vi "StationMeteo.vi"() -> ()   [LabVIEW 2018]
uses:
  <vilib>/Instr/_visa.llb/VISA Configure Serial Port (Instr).vi
panel:
  out "Nombre mesures":dbl
  out "Moyenne 3":dbl
  out "Maximum 3":dbl
  out "Minimum 3":dbl
  out "Moyenne 2":dbl
  out "Maximum 2":dbl
  out "Minimum 2":dbl
  out "Moyenne":dbl
  out "Maximum":dbl
  out "Minimum":dbl
  in  "Nom du fichier":string
  in  "Seléctionner un répertoire":bool
  out "Répertoire":path
  in  "Export valeurs":bool
  out "?":bool
  out "CSV string":string
  in  "En marche":bool
  out "Waveform Graph":dbl[](graph)
  out "boucle":dbl[](array[numeric])
  out "temperature test":dbl[](array[numeric])
  out "XY Graph":T1(graph)
  out "Humidité":dbl(graph)
  out "Pression":dbl(graph)
  out "Température":dbl(graph)
  out "Humidité temps réel":dbl
  out "Pression temps réel":dbl
  out "Température temps réel":dbl
  out "Chaîne":string
  in  "stop":bool
  in  "Nom de ressource VISA":refnum<visa-resource-name>
  # "1. Brancher la carte Arduino sur un port USB\n2. Choisir le port COM de la carte dans la liste déroulante \"Nom de ressource VISA\"\n3. Lancer le programme"
  # "Contrôles de la station météo"
  # "Valeurs particulières"
  # "Valeurs particulières"
  # "Sauvegardes des mesures en CSV"
  # "Valeurs particulières"
  # ".csv"
  # "Fichier global"
  # "Fichier séparé"
  # "Fichier séparé rajoute un -numéro à la fin \nnom de fichier. Ex: releve-5.csv\nFichier global rajoute un -global à la fin \ndu nom de fichier. Ex: releve-global.csv"
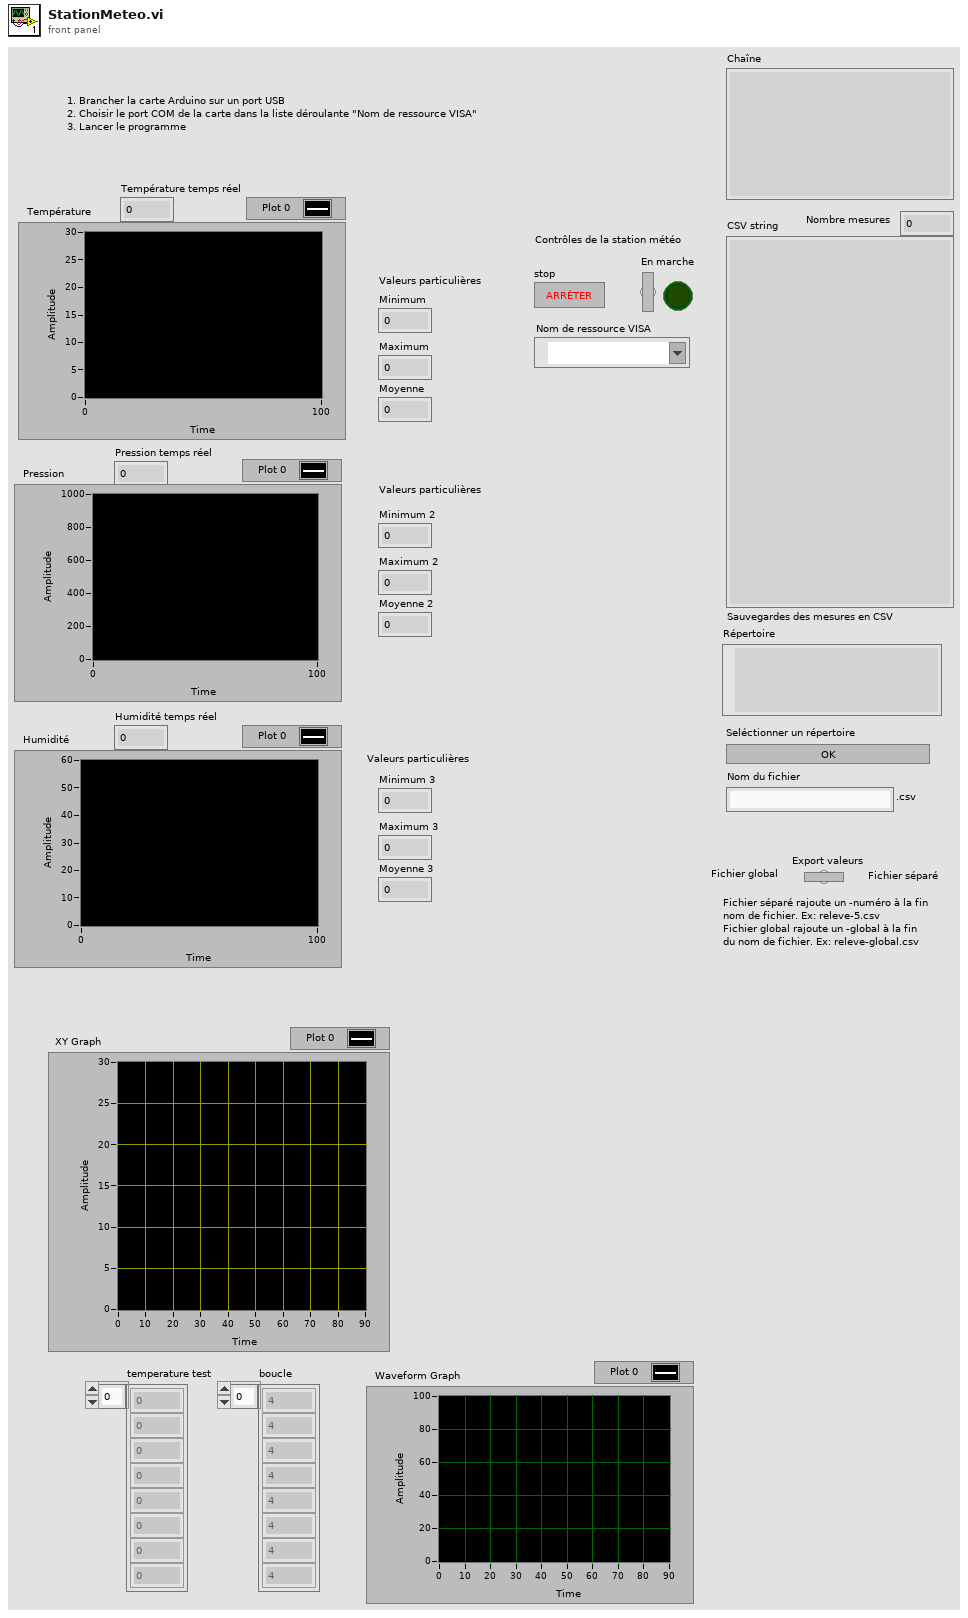
[diagram p1: front panel]
types:
  T1 = cluster{"temperature test":dbl[], "boucle":dbl[]}
  T2 = cluster{"boucle":dbl[], "temperature test":dbl[]}
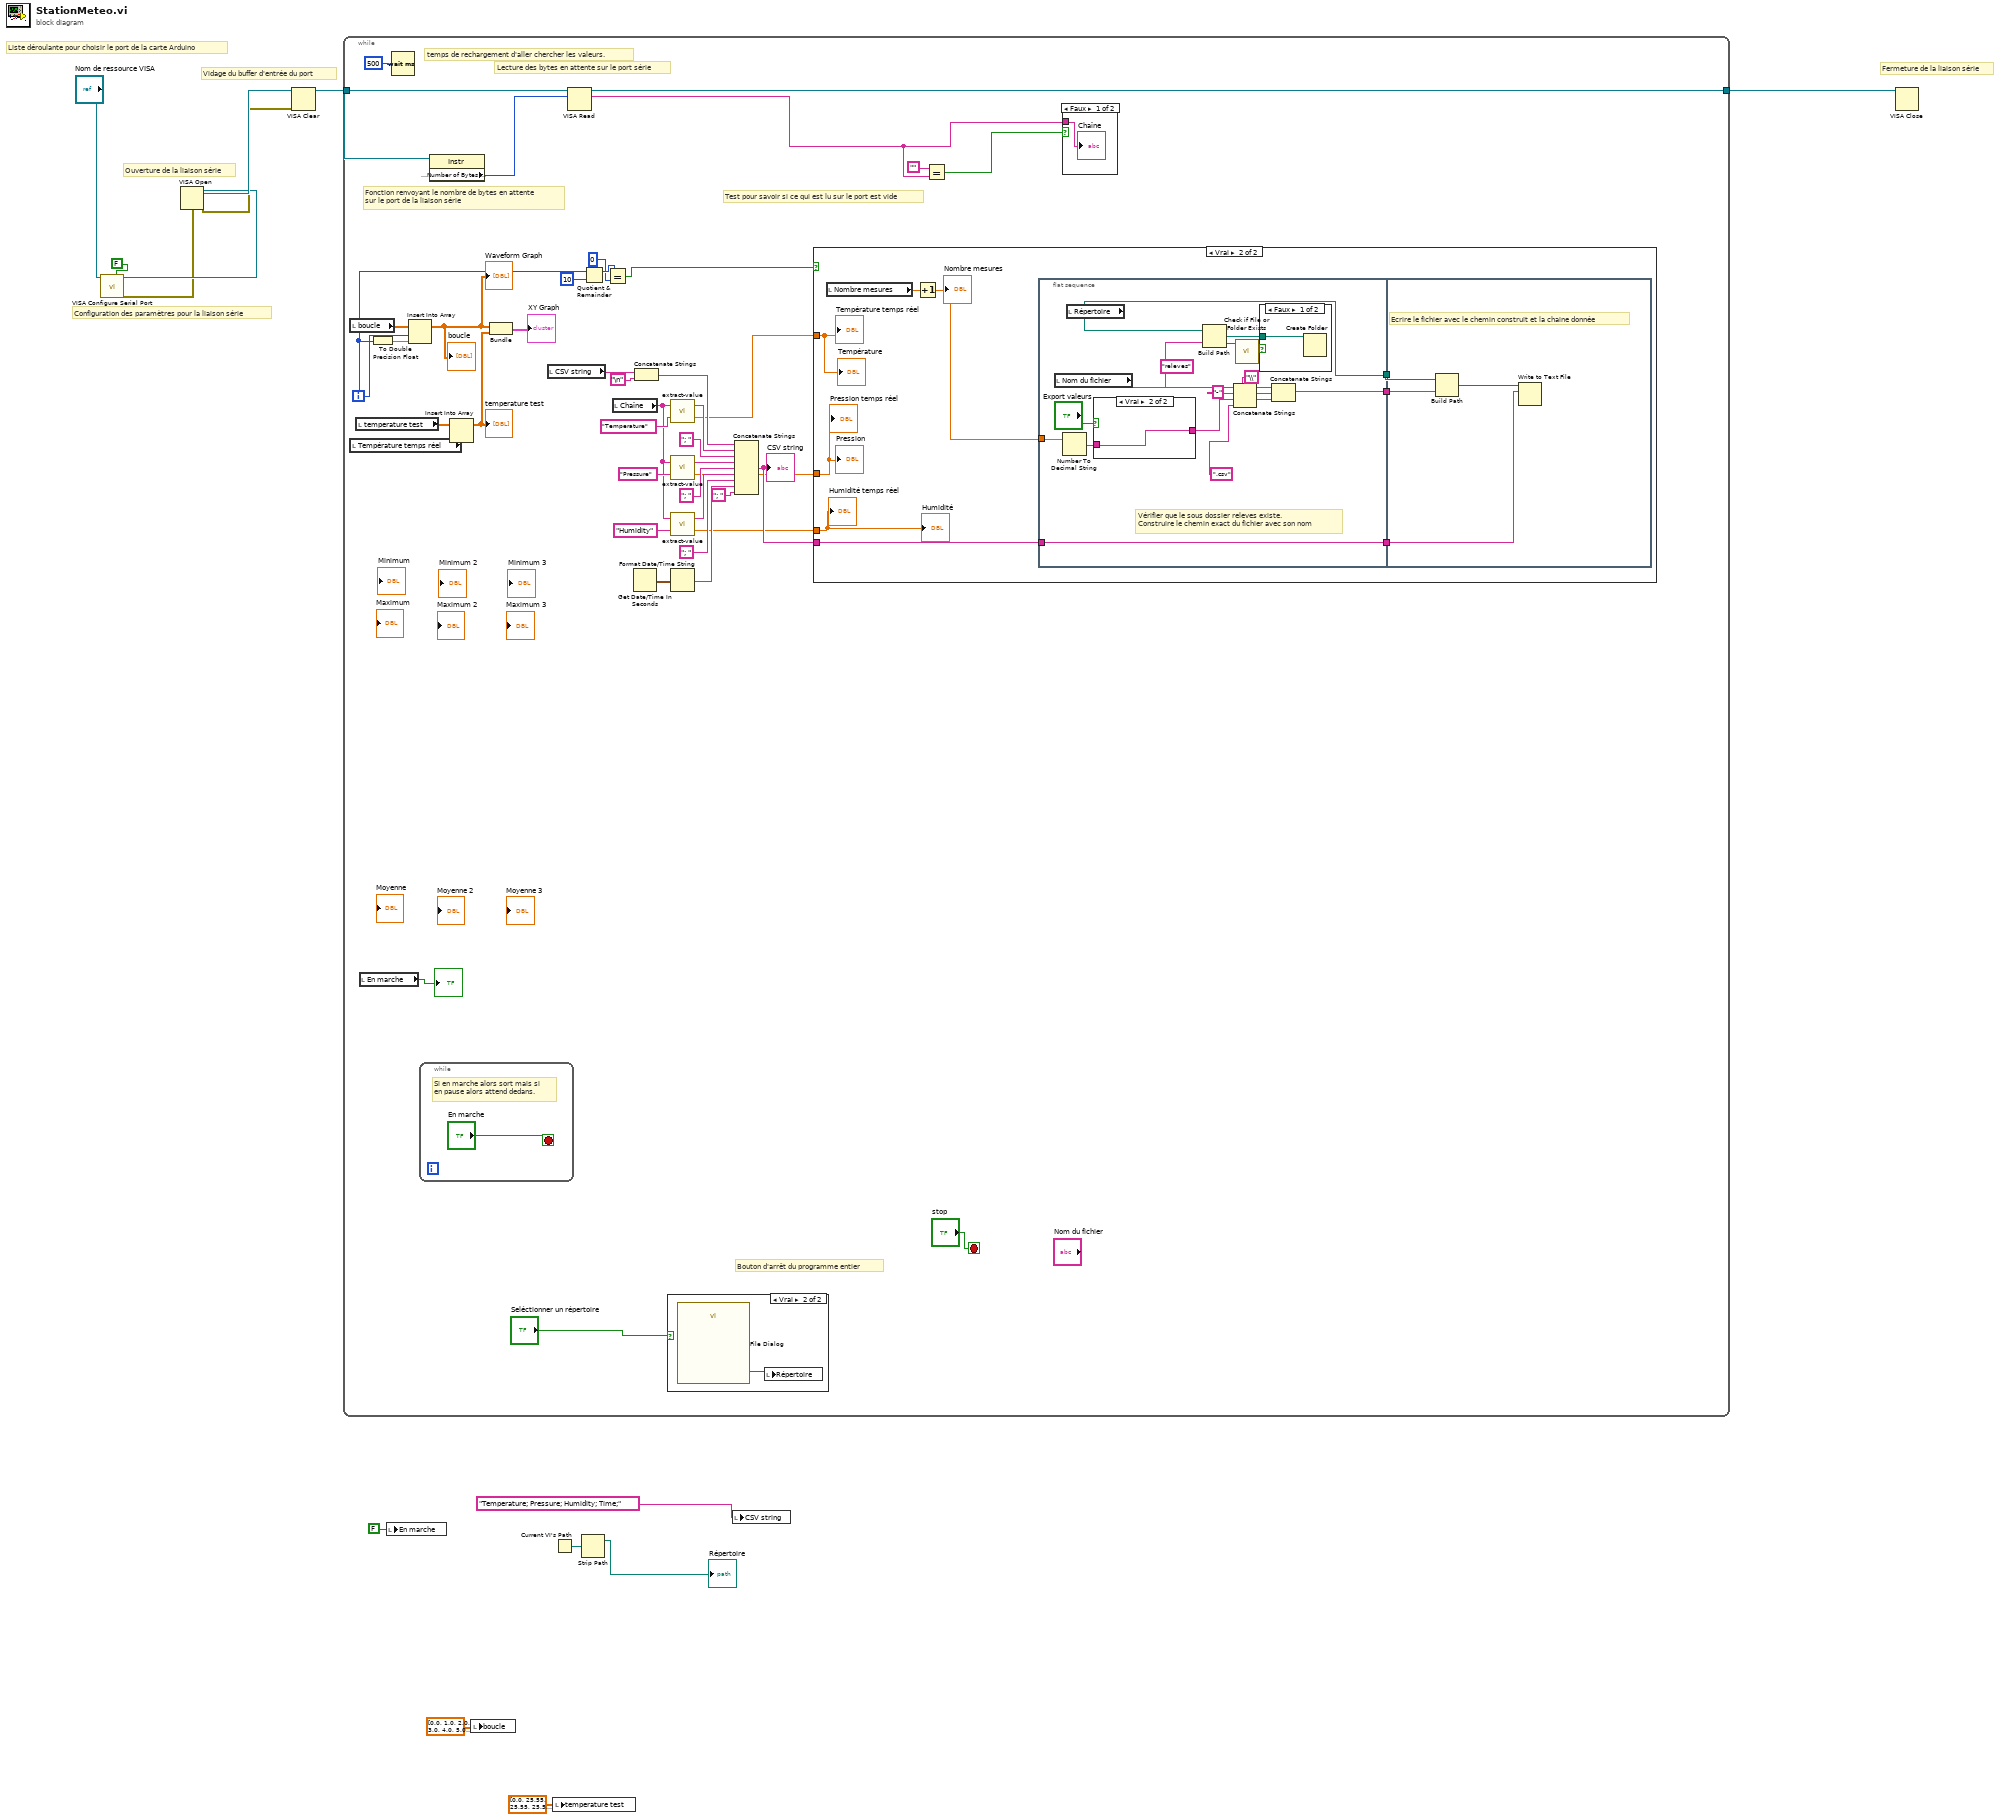
[diagram p0: block diagram]
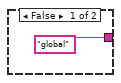
[diagram p3: hidden frame]
diagram:
  # "Vidage du buffer d'entrée du port"
  # "Ouverture de la liaison série"
  # "Configuration des paramètres pour la liaison série"
  # "Liste déroulante pour choisir le port de la carte Arduino"
  # "Fermeture de la liaison série"
  n1 = call-poly "VISA Configure Serial Port"("VISA resource name"="Nom de ressource VISA", "Enable Termination\nChar (T)"=FALSE ("Enable Termination\nChar (T)")) -> ("VISA resource name out"=w11:refnum<visa-resource-name>, "error out"=w9:errorcluster)  [unwired: 12 in]
  n2 = VISA Open(error in (no error)=w9, VISA resource name=w11) -> (VISA resource name=w13:refnum<visa-resource-name>, error out=w8:errorcluster)  [unwired: 3 in]
  n3 = VISA Clear(VISA resource name=w13, error in (no error)=w8) -> (VISA resource name out=w12:refnum<visa-resource-name>)  [unwired: 1 out]
  n4 = while {
    tunnel: w12 -> [w55]
    tunnel: [w53] -> w7
    i -> [w15]
    stop <- "stop" stop-if-true
    # "temps de rechargement d'aller chercher les valeurs."
    # "Lecture des bytes en attente sur le port série"
    # "Fonction renvoyant le nombre de bytes en attente\nsur le port de la liaison série"
    # "Test pour savoir si ce qui est lu sur le port est vide"
    # "Bouton d'arrêt du programme entier"
    n5 = local read "boucle"() -> (w47:dbl[])
    n6 = local read "Température temps réel"() -> (w48:dbl)
    n7 = local read "temperature test"() -> (w44:dbl[])
    n8 = local read "En marche"() -> (→"?":bool)
    n9 = To Double Precision Float(number=w15) -> (double precision float=w46:dbl)
    n10 = Wait (ms)(milliseconds to wait=u32 500 ("attente (ms)")) -> ()  [unwired: 1 out]
    n11 = Insert Into Array(array=w47, index=w15, new element=w46) -> (w42:dbl[])
    "boucle" <- w42
    "Waveform Graph" <- w42
    n12 = while {
      stop <- "En marche" stop-if-true
      # "Si en marche alors sort mais si \nen pause alors attend dedans."
    }
    n13 = property class="Instr"(reference=w55) -> ("Serial Settings:Number of Bytes at Serial Port"=w54:u32)  [unwired: 1 in, 2 out]
    n14 = Insert Into Array(array=w44, new element=w48) -> (w43:dbl[])  [unwired: 1 in]
    "temperature test" <- w43
    n15 = Bundle("boucle"=w42, "temperature test"=w43) -> (→"XY Graph":T2)  [unwired: 1 in]
    n16 = local read "CSV string"() -> (w38:string)
    n17 = VISA Read(VISA resource name=w55, byte count=w54) -> (VISA resource name out=w53:refnum<visa-resource-name>, read buffer=w49:string)  [unwired: 1 in, 2 out]
    n18 = Quotient & Remainder(x=w15, y=10) -> (x-y*floor(x/y)=w23:i32)  [unwired: 1 out]
    n19 = Equal?(x=w23, y=0) -> (x = y?=w21:bool)
    n20 = local read "Chaîne"() -> (w31:string)
    n21 = Get Date/Time In Seconds() -> (seconds since 1Jan1904=w27:timestamp)
    n22 = Concatenate Strings(w38, "\n") -> (w20:string)
    n23 = case shown="Vrai" "Seléctionner un répertoire" {
      frame False {
      }
      frame True {
        n24 = call "File Dialog"() -> ("selected path"=w88:path)  [unwired: 12 in, 3 out]
        n25 = local write "Répertoire"(w88) -> ()
      }
    }
    n26 = call "extract-value.vi"("Variable"="Temperature", "Chaine contenant valeur"=w31) -> ("Valeur"=w18:dbl, "Valeur en string"=w33:string)
    n27 = call "extract-value.vi"("Variable"="Pressure", "Chaine contenant valeur"=w31) -> ("Valeur"=w17:dbl, "Valeur en string"=w35:string)
    n28 = call "extract-value.vi"("Variable"="Humidity", "Chaine contenant valeur"=w31) -> ("Valeur"=w16:dbl, "Valeur en string"=w30:string)
    n29 = Format Date/Time String(seconds (now)=w27) -> (date/time string=w26:string)  [unwired: 2 in]
    n30 = Concatenate Strings(w20, w33, "; ", w35, "; ", w30, "; ", w26, "; ") -> (w19:string)
    "CSV string" <- w19
    n31 = case shown="Vrai" w21 {
      tunnel: w19 -> [_ w61]
      tunnel: w18 -> [_ w60]
      tunnel: w17 -> [_ w59]
      tunnel: w16 -> [_ w58]
      frame False {
      }
      frame True {
        n32 = local read "Nombre mesures"() -> (w65:dbl)
        n33 = Increment(x=w65) -> (x+1=w57:dbl)
        "Nombre mesures" <- w57
        n34 = flat-sequence {
          tunnel: [w74] -> w64
          tunnel: [w73] -> w63
          tunnel: [w67] -> w62
          tunnel: w61 -> [w67]
          tunnel: w57 -> [w66]
          tunnel: w64 -> [w87]
          tunnel: w63 -> [w85]
          tunnel: w62 -> [w84]
          frame #0 {
            w77 = "releves" ("name or relative path")
            # "Vérifier que le sous dossier releves existe.\nConstruire le chemin exact du fichier avec son nom"
            n35 = local read "Nom du fichier"() -> (w72:string)
            n36 = Number To Decimal String(number=w66) -> (decimal integer string=w69:string)  [unwired: 1 in]
            n37 = local read "Répertoire"() -> (w73:path)
            n38 = case shown="Vrai" "Export valeurs" {
              tunnel: w69 -> [_ w82]
              tunnel: ["global" w82] -> w68
              frame False {
              }
              frame True {
              }
            }
            n39 = Build Path(base path=w73, name or relative path=w77) -> (appended path=w79:path)
            n40 = Concatenate Strings(w72, "-" ("string"), w68, ".csv" ("string")) -> (w75:string)
            n41 = call <vilib>:"Check if File or Folder Exists.vi"("path"=w79) -> ("file or folder exists?"=w80:bool)  [unwired: 8 in, 2 out]
            n42 = case shown="Faux" w80 {
              tunnel: w79 -> [w83 _]
              frame False {
                n43 = Create Folder(path (use dialog)=w83) -> ()  [unwired: 2 in, 3 out]
              }
              frame True {
              }
            }
            n44 = Concatenate Strings(w77, "\\" ("string"), w75) -> (w74:string)
          }
          frame #1 {
            # "Ecrire le fichier avec le chemin construit et la chaine donnée"
            n45 = Build Path(base path=w85, name or relative path=w87) -> (appended path=w86:path)
            n46 = Write to Text File(file (use dialog)=w86, text=w84) -> ()  [unwired: 2 in, 3 out]
          }
        }
        "Température" <- w60
        "Température temps réel" <- w60
        "Pression temps réel" <- w59
        "Humidité temps réel" <- w58
        "Pression" <- w59
        "Humidité" <- w58
      }
    }
    n47 = Equal?(x="", y=w49) -> (x = y?=w50:bool)
    n48 = case shown="Faux" w50 {
      tunnel: w49 -> [w90 _]
      frame False {
        "Chaîne" <- w90
      }
      frame True {
      }
    }
  }
  n49 = local write "En marche"(FALSE ("En marche")) -> ()
  n50 = local write "boucle"(dbl[] [0.0, 1.0, 2.0, 3.0, 4.0, 5.0, 6.0, 7.0, 8.0, 9.0, 10.0, 11.0, 12.0, 13.0, 14.0, 15.0, 16.0, 17.0, 18.0, 19.0, 20.0, 21.0, 22.0, 23.0, 24.0, 25.0, 26.0, 27.0, 28.0, 29.0, 30.0, 31.0, 32.0, 33.0, 34.0, 35.0, 36.0, 37.0, 38.0, 39.0, 40.0, 41.0, 42.0, 43.0, 44.0, 45.0, 46.0, 47.0, 48.0, 49.0, 50.0, 51.0, 52.0, 53.0, 54.0, 55.0, 56.0, 57.0, 58.0, 59.0, 60.0, 61.0, 62.0, 63.0, 64.0, 65.0, 66.0, 67.0, 68.0, 69.0, 70.0, 71.0, 72.0, 73.0, 74.0, 75.0, 76.0, 77.0, 78.0, 79.0, 80.0, 81.0, 82.0, 83.0, 84.0, 85.0, 0.0] ("boucle")) -> ()
  n51 = local write "temperature test"(dbl[] [0.0, 25.55, 25.55, 25.55, 25.55, 25.55, 25.55, 25.55, 25.55, 25.55, 25.55, 25.55, 25.48, 25.48, 25.48, 25.48, 25.48, 25.48, 25.48, 25.48, 25.48, 25.48, 25.48, 25.48, 25.48, 25.48, 25.48, 25.48, 25.48, 25.48, 25.48, 25.48, 25.47, 25.47, 25.47, 25.47, 25.47, 25.47, 25.47, 25.47, 25.47, 25.47, 25.47, 25.47, 25.47, 25.47, 25.47, 25.47, 25.47, 25.47, 25.47, 25.47, 25.48, 25.48, 25.48, 25.48, 25.48, 25.48, 25.48, 25.48, 25.48, 25.48, 25.48, 25.48, 25.48, 25.48, 25.48, 25.48, 25.48, 25.48, 25.48, 25.48, 25.48, 25.48, 25.48, 25.48, 25.48, 25.48, 25.48, 25.48, 25.48, 25.48, 25.5, 25.5, 25.5, 25.5, 25.5] ("temperature test")) -> ()
  n52 = Current VI's Path() -> (path=w2:path)
  n53 = Strip Path(path=w2) -> (stripped path=→"Répertoire":path)  [unwired: 1 out]
  n54 = local write "CSV string"("Temperature; Pressure; Humidity; Time;") -> ()
  n55 = VISA Close(VISA resource name=w7) -> ()  [unwired: 1 in, 1 out]
